vi "ZMC Get Time Out.vi"(8 "error in (no error)":errorcluster caption="错误输入（无错误）", 10 "ptimems":u32, 11 "handle":u32) -> (0 "error out":errorcluster caption="错误输出", 1 "function return":i32, 2 "ptimems out":u32, 3 "handle out":u32)   [LabVIEW 2015, in "zauxdll.lvlib"]
doc: "int32 __stdcall ZMC_GetTimeOut(ZMC_HANDLE handle, uint32* ptimems);"
uses:
  zauxdll.lvlib
  zmotion.dll
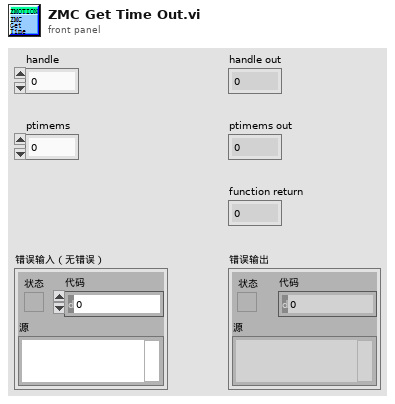
[diagram p1: front panel]
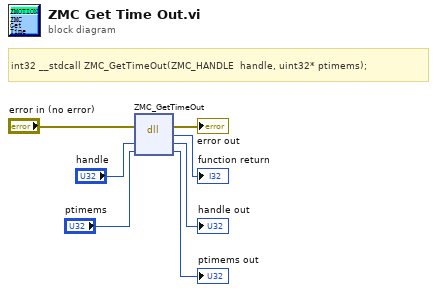
[diagram p0: block diagram]
diagram:
  # "int32 __stdcall ZMC_GetTimeOut(ZMC_HANDLE  handle, uint32* ptimems);"
  n1 = dll-call lib="C:/Users/VIC/Desktop/GOGORO_SA/system/LLB/zmotion/zaux/zmotion.*" fn="ZMC_GetTimeOut"(error in="error in (no error)", "handle"="handle", "ptimems"="ptimems") -> (error out=→"error out":errorcluster, →"function return":i32, "handle"=→"handle out":u32, "ptimems"=→"ptimems out":u32)  [unwired: 2 in, 1 out]
